vi "Handle Variable Header.vi"(8 "error in (no error)":errorcluster, 10 "Incoming Packets":u8[](array[numeric]) format="%08b", 11 "CONNECT in":refnum<class "CONNECT.lvclass">) -> (0 "error out":errorcluster, 1 "Variable Header Complete?":bool=TRUE, 2 "Remaining Packets":u8[](array[numeric]) format="%08b", 3 "CONNECT out":refnum<class "CONNECT.lvclass">)   [LabVIEW 2013, in "CONNECT.lvclass"]
uses:
  CONNECT.lvclass
  ControlPacket/ControlPacket.lvclass/ControlPacket.ctl
  ControlPacket/ControlPacket.lvclass
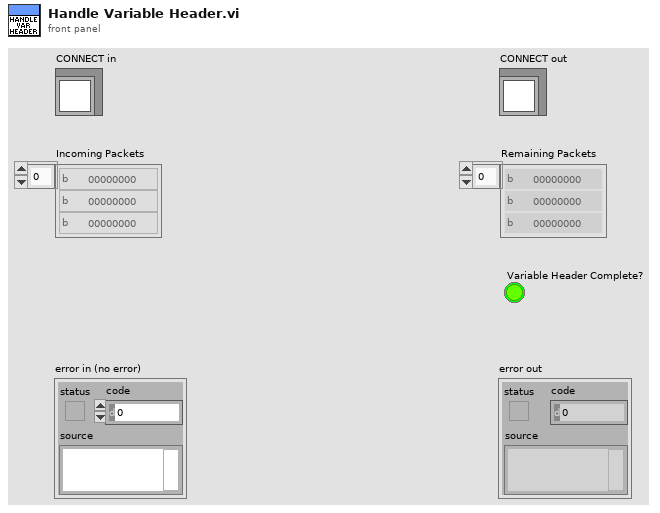
[diagram p1: front panel]
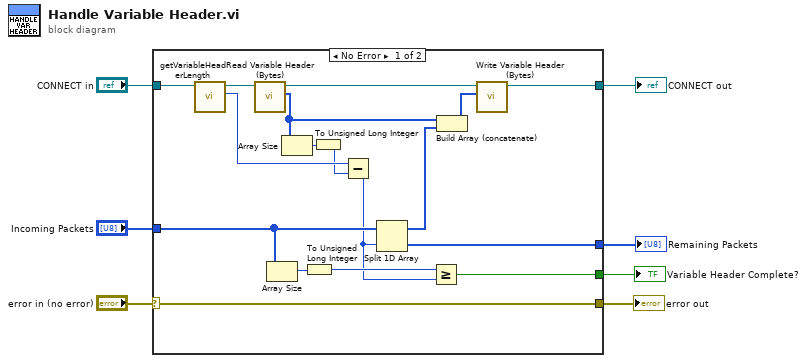
[diagram p0: block diagram]
diagram:
  n1 = case shown="No Error" "error in (no error)" {
    selector: "error in (no error)" -> [w8 w25]
    tunnel: "CONNECT in" -> [w22 w27]
    tunnel: "Incoming Packets" -> [w15 w26]
    tunnel: [w11 _] -> w5
    tunnel: [w10 w26] -> w4
    tunnel: [w9 w27] -> w3
    tunnel: [w8 w25] -> w1
    frame No Error {
      n2 = call-dynamic "getVariableHeaderLength.vi"("CONNECT in"=w22) -> ("VariableHeader size"=w17:u32, "CONNECT out"=w24:refnum<class "CONNECT.lvclass">)  [unwired: 8 in, 1 out]
      n3 = call "Read Variable Header (Bytes).vi"("ControlPacket in"=w24) -> ("Variable Header (Bytes)"=w20:u8[], "ControlPacket out"=w23:refnum<class "CONNECT.lvclass">)  [unwired: 9 in]
      n4 = Array Size(array=w15) -> (size(s)=w14:i32)
      n5 = Array Size(array=w20) -> (size(s)=w21:i32)
      n6 = To Unsigned Long Integer(number=w14) -> (unsigned 32bit integer=w13:u32)
      n7 = To Unsigned Long Integer(number=w21) -> (unsigned 32bit integer=w16:u32)
      n8 = Subtract(x=w17, y=w16) -> (x-y=w12:u32)
      n9 = Split 1D Array(array=w15, index=w12) -> (first subarray=w19:u8[], second subarray=w10:u8[])
      n10 = Greater Or Equal?(x=w13, y=w12) -> (x >= y?=w11:bool)
      n11 = Build Array (concatenate)(w20, w19) -> (w18:u8[])
      n12 = call "Write Variable Header (Bytes).vi"("Variable Header (Bytes)"=w18, "ControlPacket in"=w23) -> ("ControlPacket out"=w9:refnum<class "CONNECT.lvclass">)  [unwired: 9 in]
    }
    frame Error {
    }
  }
  "error out" <- w1
  "CONNECT out" <- w3
  "Remaining Packets" <- w4
  "Variable Header Complete?" <- w5
